vi "configureImageAcquisition.vi"(8 "error in (no error)":errorcluster, 9 "Image Binning":T1={"Vertical Binning"=1.0, "Horizontal Binning"=1.0, "SubArea Height"=0.0, "SubAreaWidth"=0.0, "Offset"=0.0, "Number of Tracks"=0.0, "Track Positions"=[], "subArea Coordinate"=[]}, 10 "Mode":T2, 11 "CameraAcquisitor in":refnum<class "CameraAcquisitor.lvclass">) -> (0 "error out":errorcluster, 3 "CameraAcquisitor out":refnum<class "CameraAcquisitor.lvclass">)   [LabVIEW 2011, in "Hardware.lvlib" / "Channels.lvlib" / "CameraAcquisitor.lvclass"]
uses:
  CameraAcquisitor.lvclass
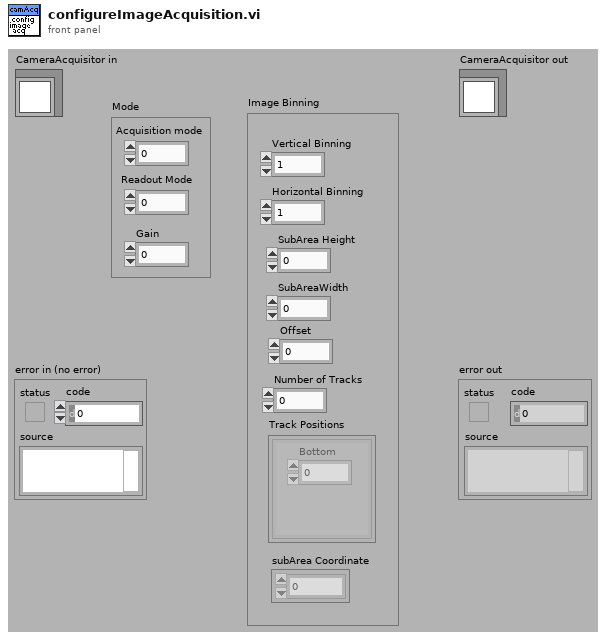
[diagram p1: front panel]
types:
  T1 = cluster{"Vertical Binning":dbl, "Horizontal Binning":dbl, "SubArea Height":dbl, "SubAreaWidth":dbl, "Offset":dbl, "Number of Tracks":dbl, "Track Positions":cluster{"Top":dbl, "Bottom ":dbl}[], "subArea Coordinate":dbl[]}
  T2 = cluster{"Acquisition mode":dbl, "Readout Mode":dbl, "Gain":dbl}
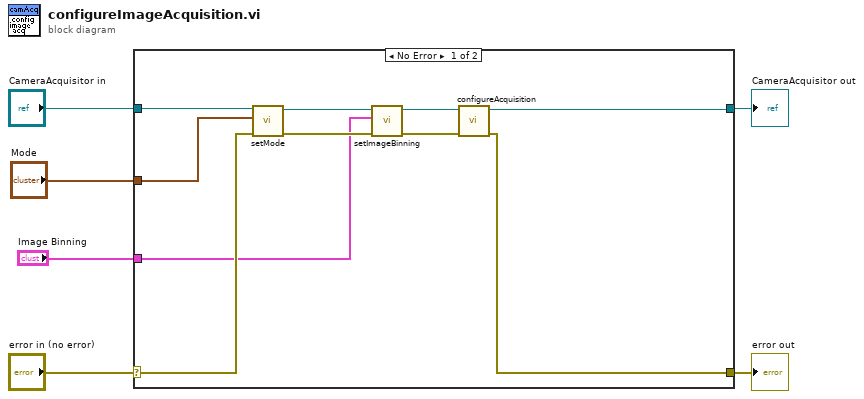
[diagram p0: block diagram]
diagram:
  n1 = case shown="No Error" "error in (no error)" {
    selector: "error in (no error)" -> [w15 w18]
    tunnel: [w9 w18] -> w5
    tunnel: [w10 w17] -> w3
    tunnel: "CameraAcquisitor in" -> [w16 w17]
    tunnel: "Mode" -> [w7 _]
    tunnel: "Image Binning" -> [w8 _]
    frame No Error {
      n2 = call-dynamic "setMode.vi"("error in (no error)"=w15, "Mode"=w7, "CameraAcquisitor.lvclass in"=w16) -> ("error out"=w13:errorcluster, "CameraAcquisitor.lvclass out"=w14:refnum<class "CameraAcquisitor.lvclass">)  [unwired: 7 in]
      n3 = call-dynamic "setImageBinning.vi"("error in (no error)"=w13, "Image Binning"=w8, "CameraAcquisitor.lvclass in"=w14) -> ("error out"=w11:errorcluster, "CameraAcquisitor.lvclass out"=w12:refnum<class "CameraAcquisitor.lvclass">)  [unwired: 7 in]
      n4 = call-dynamic "configureAcquisition.vi"("error in (no error)"=w11, "CameraAcquisitor in"=w12) -> ("error out"=w9:errorcluster, "CameraAcquisitor out"=w10:refnum<class "CameraAcquisitor.lvclass">)  [unwired: 8 in]
    }
    frame Error {
    }
  }
  "error out" <- w5
  "CameraAcquisitor out" <- w3
